vi "Set State_Measure iVIO and HV.vi"(0 "Semiconductor Module Context":T1, 1 "script name":string, 2 "Delay Time (s)":dbl=0.001 format="%#_13p", 7 "Power_Pins":string[](array[string]), 9 "Published Data Ids":string[](array[string]), 11 "error in (no error)":errorcluster) -> (15 "error out":errorcluster)   [LabVIEW 2013]
uses:
  <vilib>/NI_TestStand_SemiconductorModule/NI_TestStand_Semiconductor_Module.lvlibp/PinMap/General/SemiconductorModuleContext.ctl
  <instrlib>/niHSDIO/niHSDIO.llb/niHSDIO_ctl Trigger Script - trigID Values (Ring).ctl
  <vilib>/NI_TestStand_SemiconductorModule/NI_TestStand_Semiconductor_Module.lvlibp/PinMap/DC Power/PinsToNIDCPowerSessions.vi
  <vilib>/NI_TestStand_SemiconductorModule/NI_TestStand_Semiconductor_Module.lvlibp/PinMap/General/Publish/PublishDataDouble2D.vi
  <vilib>/NI_TestStand_SemiconductorModule/NI_TestStand_Semiconductor_Module.lvlibp
panel:
  out "HV_measurements":dbl[][](array[numeric])
  out "iVIO_measurements":dbl[][](array[numeric])
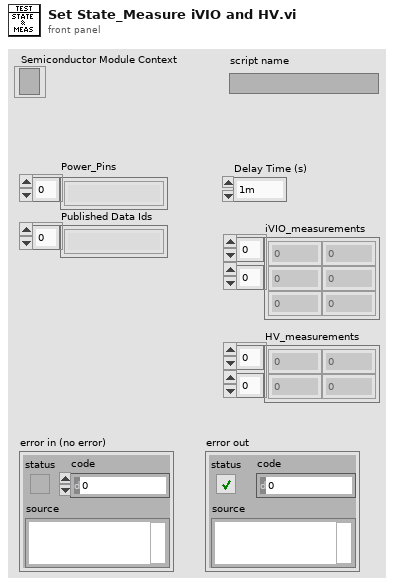
[diagram p1: front panel]
types:
  T1 = typedef "NI_TestStand_Semiconductor_Module.lvlibp/SemiconductorModuleContext.ctl" = refnum<k7>
  T2 = typedef "niHSDIO_ctl Trigger Script - trigID Values (Ring).ctl" = string
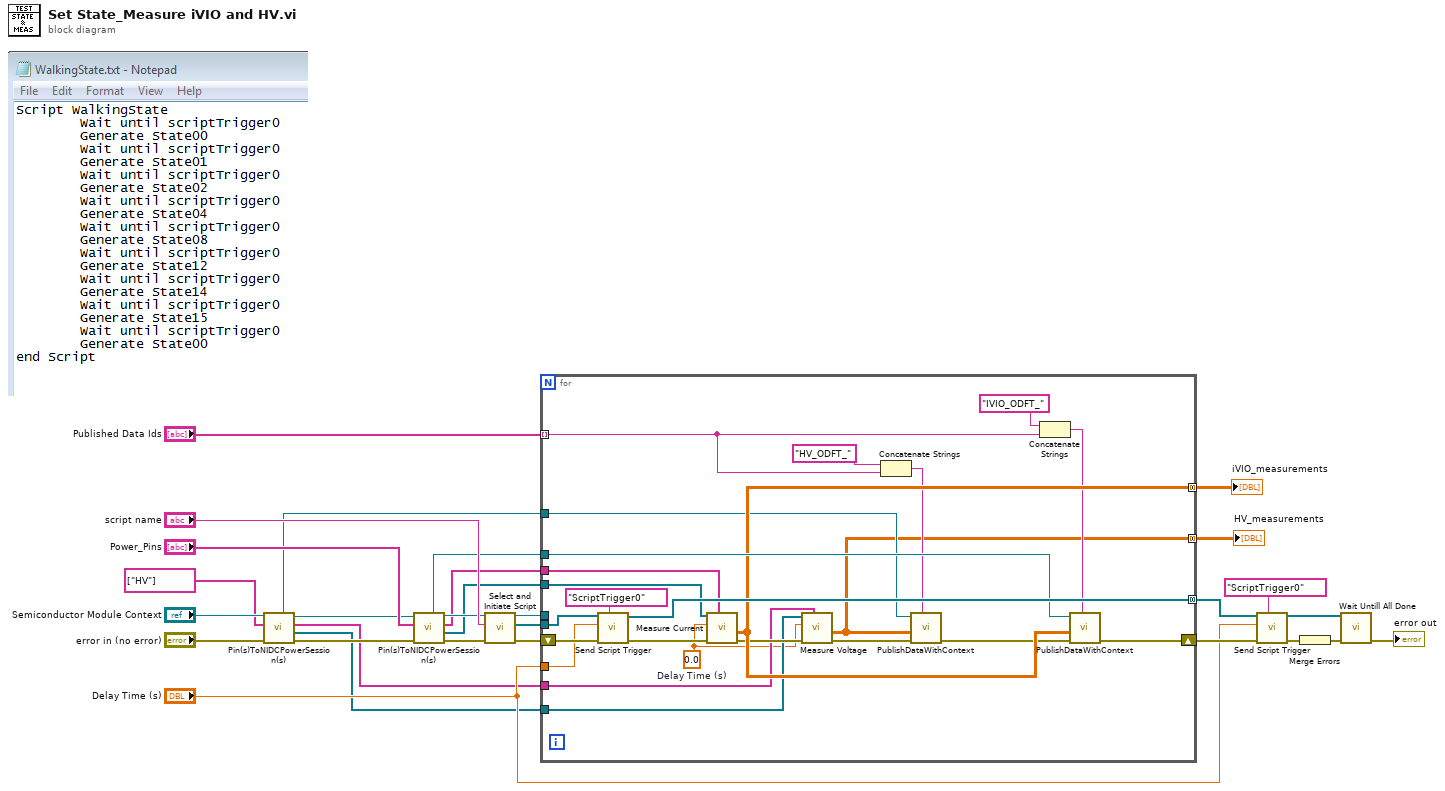
[diagram p0: block diagram]
diagram:
  n1 = call-poly <vilib>:"Pin(s)ToNIDCPowerSession(s).vi"("error in (no error)"="error in (no error)", "Pins"=string[] ["HV"], "Semiconductor Module Context"="Semiconductor Module Context") -> ("error out"=w7:errorcluster, "Instrument Sessions"=w2:refnum<k15>[], "Channel Lists"=w1:string[], "Semiconductor Module Context Out"=w5:T1, "Pin Query Context"=w3:refnum<class "MultiplePinMultipleSessionQueryContext.lvclass">)  [unwired: 4 in]
  n2 = call-poly <vilib>:"Pin(s)ToNIDCPowerSession(s).vi"("error in (no error)"=w7, "Pins"="Power_Pins", "Semiconductor Module Context"=w5) -> ("error out"=w18:errorcluster, "Instrument Sessions"=w15:refnum<k15>[], "Channel Lists"=w14:string[], "Semiconductor Module Context Out"=w17:T1, "Pin Query Context"=w12:refnum<class "MultiplePinMultipleSessionQueryContext.lvclass">)  [unwired: 4 in]
  n3 = call "Select and Initiate Script.vi"("error in (no error)"=w18, "script name"="script name", "Semiconductor Module Context"=w17) -> ("error out"=w29:errorcluster, "HSDIO GEN Sessions Out"=w28:refnum<k15>[], "Semiconductor Module Context Out"=w26:T1)  [unwired: 6 in]
  n4 = for {
    tunnel: w28 -> [w52]
    tunnel: w26 -> [_]
    tunnel: "Published Data Ids" -> [w36] mode=indexing
    tunnel: [w50] -> w20 mode=concatenating
    shift-right: [w47] -> w13
    shift-left: w29 -> [w53]
    tunnel: w15 -> [w48]
    tunnel: w14 -> [w49]
    tunnel: w12 -> [w46]
    tunnel: [w45] -> w11 mode=concatenating
    tunnel: "Delay Time (s)" -> [w41]
    tunnel: [w31] -> w9 mode=concatenating
    tunnel: w3 -> [w39]
    tunnel: w2 -> [w32]
    tunnel: w1 -> [w33]
    w30 = 0.0  # Delay Time (s)
    n5 = call "Send Script Trigger.vi"("trigger id (script trigger 0)"=T2 "ScriptTrigger0", "error in (no error)"=w53, "Delay Time (s)"=w41, "HSDIO Sessions In"=w52) -> ("error out"=w42:errorcluster, "HSDIO Sessions Out"=w50:refnum<k15>[])  [unwired: 6 in]
    n6 = call "Measure Current.vi"("Channel Lists"=w49, "error in (no error)"=w42, "Delay Time (s)"=w30, "DCPower Sessions In"=w48) -> ("error out"=w34:errorcluster, "current measurements"=w45:dbl[][])  [unwired: 5 in, 1 out]
    n7 = call "Measure Voltage.vi"("Channel Lists"=w33, "error in (no error)"=w34, "Delay Time (s)"=w30, "DCPower Sessions In"=w32) -> ("error out"=w35:errorcluster, "Voltage measurements"=w31:dbl[][])  [unwired: 5 in, 1 out]
    n8 = Concatenate Strings("HV_ODFT_" ("Published Data Id"), w36) -> (w37:string)
    n9 = call-poly <vilib>:"PublishDataWithContext.vi"("Published Data Id"=w37, "error in (no error)"=w35, "Data In"=w31, "Pin Query Context"=w39) -> ("error out"=w40:errorcluster)  [unwired: 6 in, 1 out]
    n10 = Concatenate Strings("IVIO_ODFT_" ("Published Data Id"), w36) -> (w44:string)
    n11 = call-poly <vilib>:"PublishDataWithContext.vi"("Published Data Id"=w44, "error in (no error)"=w40, "Data In"=w45, "Pin Query Context"=w46) -> ("error out"=w47:errorcluster)  [unwired: 6 in, 1 out]
  }
  "iVIO_measurements" <- w11
  "HV_measurements" <- w9
  n12 = call "Send Script Trigger.vi"("trigger id (script trigger 0)"=T2 "ScriptTrigger0", "error in (no error)"=w13, "Delay Time (s)"="Delay Time (s)", "HSDIO Sessions In"=w20) -> ("error out"=w21:errorcluster, "HSDIO Sessions Out"=w19:refnum<k15>[])  [unwired: 6 in]
  n13 = Merge Errors(w21) -> (w24:errorcluster)
  n14 = call "Wait Untill All Done.vi"("error in (no error)"=w24, "HSDIO Sessions In"=w19) -> ("error out"=→"error out":errorcluster)  [unwired: 8 in, 1 out]
